vi "RT Driver VI.vi"(7 "Operation":T1, 11 "Device Reference in":T2 format="%.0x") -> (0 "Error Code":i32)   [LabVIEW 2016, in "DDS Custom Device Engine.lvlib"]
uses:
  DDS Custom Device Engine.lvlib
  <vilib>/NI Veristand/Custom Device API/Custom Device Item Ref.ctl
  <vilib>/NI Veristand/Custom Device API/Hardware Interface Driver VI Operation.ctl
  Shared/Compiled.Settings.ctl
  Shared/WriterReaderConfiguration.ctl
  Shared/Advanced DDS Configuration.ctl
  Shared/key Enum.ctl
  <vilib>/RTI DDS Toolkit/Types/RTI DDS ContentFilteredTopic Info.ctl
  RTStateVariables.ctl
  <vilib>/ni/NIVS Inline Async API/_VS Inline Async API/VS Inline Async API/VS Inline Async API.lvclass
  Shared/MyTopic ComplexType.ctl
  <vilib>/ni/NIVS Inline Async API/_VS Inline Async API/VS Inline Async API/VS Inline Async API.lvclass/VS Inline Async API.ctl
  <vilib>/ni/NIVS Inline Async API/_Data Access Engine/Data Access Engine/Data Access Engine.lvclass/Data Access Engine.ctl
  <vilib>/ni/NIVS Inline Async API/_Data Access Engine/Access Type Classes/Write/Write.lvclass/Write.ctl
  <vilib>/ni/NIVS Inline Async API/_Data Access Engine/Access Type Classes/ReadWrite/ReadWrite.lvclass/ReadWrite.ctl
  <vilib>/ni/NIVS Inline Async API/_Data Access Engine/Access Type Classes/Read/Read.lvclass/Read.ctl
  <vilib>/ni/NIVS Inline Async API/_Data Access Engine/Data Access Engine/Methods/Data.Engine.Read Data from HW.vi
  <vilib>/ni/NIVS Inline Async API/_VS Inline Async API/Error Handling Process/SubVIs/Error.GetError.vi
  <vilib>/ni/NIVS Inline Async API/_Data Access Engine/Data Access Engine/Methods/Data.Engine.Write Data to HW.vi
  <vilib>/ni/NIVS Inline Async API/_Data Access Engine/Access Type Classes/ReadWrite/ReadWrite.EngineData.vi
  <vilib>/ni/NIVS Inline Async API/_Data Access Engine/Access Type Classes/Write/Write.EngineData.vi
  <vilib>/ni/NIVS Inline Async API/_Data Access Engine/Access Type Classes/Read/Read.EngineData.vi
  <vilib>/NI Veristand/Custom Device API/NI VeriStand - Get Channel Value by Data Reference.vi
  <vilib>/NI Veristand/Custom Device API/NI VeriStand - Set Channel Value by Data Reference.vi
  <vilib>/NI Veristand/Custom Device API/NI VeriStand - Get Channel Values by Block Data Reference.vi
  Shared/Constants.vi
  <vilib>/NI Veristand/Custom Device API/Get Item Property (Variant).vi
  MyTopic ComplexType Writer.vi
  <vilib>/NI Veristand/Custom Device API/Global Data Refs.vi
  <vilib>/NI VeriStand/Custom Device API/Custom Device API.lvlib
  <vilib>/NI VeriStand/Custom Device Tools/Custom Device Utility Library/Custom Device Utility Library.lvlib
  Shared/DDS Custom Device Shared.lvlib
  <vilib>/RTI DDS Toolkit/Library/LVDDS_library.lvlib
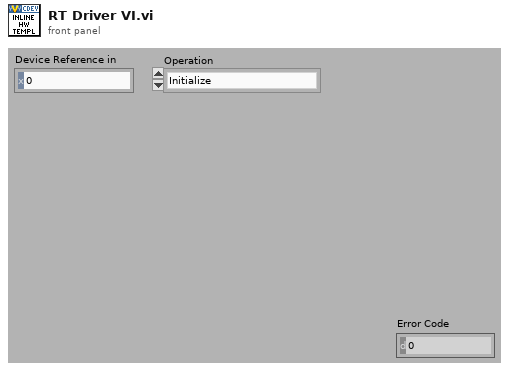
[diagram p1: front panel]
types:
  T1 = typedef "Custom Device API.lvlib/Hardware Interface Driver VI Operation.ctl" = enum16{"Initialize", "Start", "Read Data from HW", "Write Data to HW", "Close"}
  T2 = typedef "Custom Device API.lvlib/Custom Device Item Ref.ctl" = u64
  T3 = typedef "DDS Custom Device Engine.lvlib/RTStateVariables.ctl" = cluster{"Async":refnum<class "VS Inline Async API.lvclass">, "Settings":T4, "complexType":T9}
  T4 = typedef "DDS Custom Device Shared.lvlib/Compiled.Settings.ctl" = cluster{"Name":string, "Topics":T5[]}
  T5 = typedef "DDS Custom Device Shared.lvlib/WriterReaderConfiguration.ctl" = cluster{"Topic Name":string, "Domain Id":u32, "Advanced Configuration":T6}
  T6 = typedef "DDS Custom Device Shared.lvlib/Advanced DDS Configuration.ctl" = cluster{"typeName":string, "key Name":T7, "domainParticipantQoSProfile":string, "dataWriterQoSProfile":string, "forceArrayMapping?":bool, "forceUnboundedString?":bool, "forceExclusiveReader?":bool, "forceRead? (only ExclusiveReader)":bool, "ContentFilteredTopic Info":T8}
  T7 = typedef "DDS Custom Device Shared.lvlib/key Enum.ctl" = enum16{"<none>", "I32_Num", "I64_Num", "U16_Num", "innercluster.Sgl_Num", "innercluster.Boolean"}
  T8 = typedef "LVDDS_library.lvlib/RTI DDS ContentFilteredTopic Info.ctl" = cluster{"Filter Type":string, "ContentFilteredTopic Name":string, "Filter Expression":string}
  T9 = typedef "DDS Custom Device Shared.lvlib/MyTopic ComplexType.ctl" = cluster{"I32_Num":i32, "I64_Num":i64, "U16_Num":u16, "Sgl_Array":sgl[], "innercluster":cluster{"Sgl_Num":sgl, "Boolean":bool}}
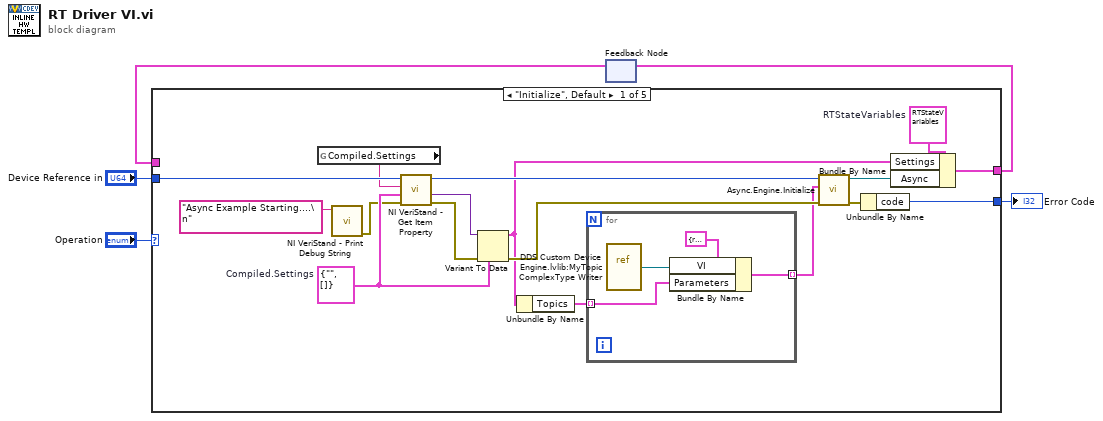
[diagram p0: block diagram]
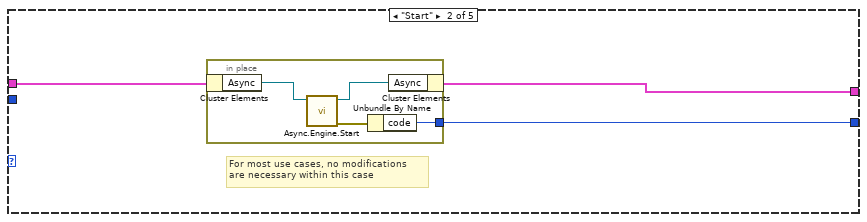
[diagram p2: hidden frame]
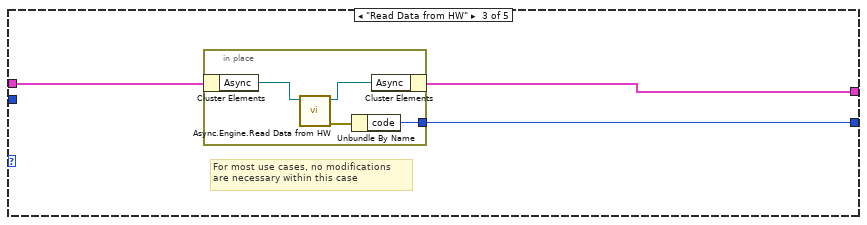
[diagram p3: hidden frame]
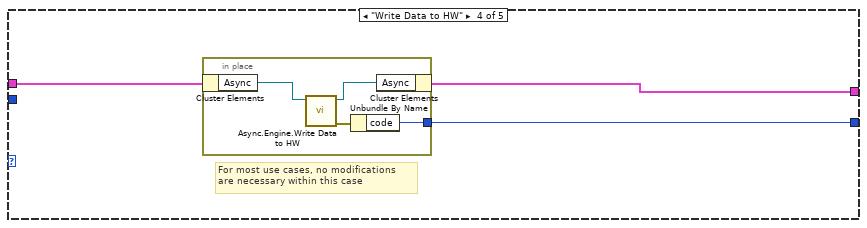
[diagram p4: hidden frame]
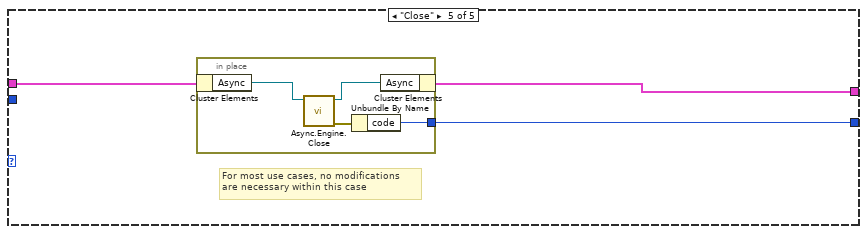
[diagram p5: hidden frame]
diagram:
  n1 = feedback #1() -> (w3:T3)  [unwired: 1 out]
  n2 = case shown="\"Initialize\", Default" "Operation" {
    tunnel: [w20 w28 w34 w41 w49] -> w4
    tunnel: w3 -> [_ w29 w36 w42 w50]
    tunnel: "Device Reference in" -> [w19 _ _ _ _]
    tunnel: [w22 w27 w35 w43 w48] -> w1
    frame "Initialize", Default {
      w13 = T3 {"Async"=refnum, "Settings"={"Name"="", "Topics"=[]}, "complexType"={"I32_Num"=0, "I64_Num"=0, "U16_Num"=0, "Sgl_Array"=[1.0, 1.0, 1.0, 1.0], "innercluster"={"Sgl_Num"=0.0, "Boolean"=FALSE}}}  # RTStateVariables
      w14 = T4 {"Name"="", "Topics"=[]}  # Compiled.Settings
      n3 = global read "Constants.vi" "Compiled.Settings"() -> (w16:string)
      n4 = call <vilib>:"NI VeriStand - Print Debug String.vi"("Message"="Async Example Starting....\n") -> ("error out"=w10:errorcluster)  [unwired: 10 in]
      n5 = call-poly <vilib>:"NI VeriStand - Get Item Property.vi"("error in (no error)"=w10, "Default Value"=w14, "Property Name"=w16, "Item Ref in"=w19) -> ("error out"=w18:errorcluster, "Value"=w17:variant, "Item Ref out"=w11:T2)  [unwired: 4 in, 1 out]
      n6 = Variant To Data(error in=w18, type=w14, Variant=w17) -> (data=w8:T4, error out=w12:errorcluster)
      n7 = Unbundle By Name(w8) -> ("Topics"=w7:T5[])
      n8 = for {
        tunnel: w7 -> [w24] mode=indexing
        tunnel: [w23] -> w6 mode=indexing
        n9 = vi-ref "DDS Custom Device Engine.lvlib:MyTopic ComplexType Writer.vi"() -> (w25:refnum<vi>)
        n10 = Bundle By Name(cluster=cluster{"VI":refnum<vi>, "Parameters":variant} {"VI"=refnum, "Parameters"=variant} ("Process"), "VI"=w25, "Parameters"=w24) -> (w23:cluster{"VI":refnum<vi>, "Parameters":variant})
      }
      n11 = call <vilib>:"Async.Engine.Initialize.vi"("error in (no error)"=w12, "Processes"=w6, "Custom Device Ref"=w11) -> ("error out"=w15:errorcluster, "Async"=w21:refnum<class "VS Inline Async API.lvclass">)  [unwired: 7 in]
      n12 = Unbundle By Name(w15) -> ("code"=w22:i32)
      n13 = Bundle By Name(cluster=w13, "Settings"=w8, "Async"=w21) -> (w20:T3)
    }
    frame "Start" {
      # "For most use cases, no modifications \nare necessary within this case"
      n14 = in-place {
        in-place-border: [w30] -> w27
        n15 = in-place-cluster #2(w29) -> ("Async"=w33:refnum<class "VS Inline Async API.lvclass">)
        n16 = call <vilib>:"Async.Engine.Start.vi"("VS Inline Async API in"=w33) -> ("error out"=w31:errorcluster, "VS Inline Async API out"=w32:refnum<class "VS Inline Async API.lvclass">)  [unwired: 9 in]
        n17 = Unbundle By Name(w31) -> ("code"=w30:i32)
        n18 = in-place-cluster #2("Async"=w32) -> (w28:T3)
      }
    }
    frame "Read Data from HW" {
      # "For most use cases, no modifications \nare necessary within this case"
      n19 = in-place {
        in-place-border: [w38] -> w35
        n20 = in-place-cluster #3(w36) -> ("Async"=w40:refnum<class "VS Inline Async API.lvclass">)
        n21 = call <vilib>:"Async.Engine.Read Data from HW.vi"("Async in"=w40) -> ("error out"=w37:errorcluster, "Async out"=w39:refnum<class "VS Inline Async API.lvclass">)  [unwired: 9 in]
        n22 = Unbundle By Name(w37) -> ("code"=w38:i32)
        n23 = in-place-cluster #3("Async"=w39) -> (w34:T3)
      }
    }
    frame "Write Data to HW" {
      # "For most use cases, no modifications \nare necessary within this case"
      n24 = in-place {
        in-place-border: [w47] -> w43
        n25 = in-place-cluster #4(w42) -> ("Async"=w45:refnum<class "VS Inline Async API.lvclass">)
        n26 = call <vilib>:"Async.Engine.Write Data to HW.vi"("VS Inline Async API in"=w45) -> ("error out"=w46:errorcluster, "VS Inline Async API out"=w44:refnum<class "VS Inline Async API.lvclass">)  [unwired: 9 in]
        n27 = Unbundle By Name(w46) -> ("code"=w47:i32)
        n28 = in-place-cluster #4("Async"=w44) -> (w41:T3)
      }
    }
    frame "Close" {
      # "For most use cases, no modifications \nare necessary within this case"
      n29 = in-place {
        in-place-border: [w52] -> w48
        n30 = in-place-cluster #5(w50) -> ("Async"=w54:refnum<class "VS Inline Async API.lvclass">)
        n31 = call <vilib>:"Async.Engine.Close.vi"("Async in"=w54) -> ("error out"=w51:errorcluster, "Async out"=w53:refnum<class "VS Inline Async API.lvclass">)  [unwired: 9 in]
        n32 = Unbundle By Name(w51) -> ("code"=w52:i32)
        n33 = in-place-cluster #5("Async"=w53) -> (w49:T3)
      }
    }
  }
  "Error Code" <- w1
  n34 = feedback-in #1(w4) -> ()
